vi "Set.vi"(10 "Time Stamp":timestamp, 11 "DateTime in":refnum<class "Timestamp.lvclass">) -> (3 "DateTime out":refnum<class "Timestamp.lvclass">)   [LabVIEW 2022 SP3, in "Conditum.lvlib" / "Columns.lvlib" / "Timestamp.lvclass"]
uses:
  Timestamp.lvclass
  C:/dev/lv/illuminated-g/lv-conditum/Conditum/Columns/Type/Type.lvclass
  Type/Type.lvclass/Type.ctl
  Timestamp.lvclass/Timestamp.ctl
  Type/Type.lvclass
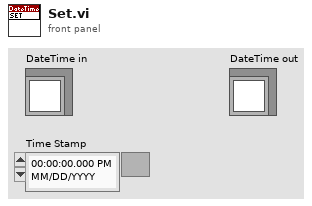
[diagram p1: front panel]
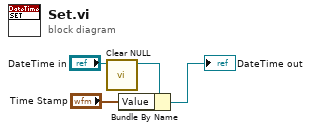
[diagram p0: block diagram]
diagram:
  n1 = call "Clear NULL.vi"("Type in"="DateTime in") -> ("Type out"=w1:refnum<class "Timestamp.lvclass">)  [unwired: 10 in]
  n2 = Bundle By Name(cluster=w1, "Value"="Time Stamp") -> (→"DateTime out":refnum<class "Timestamp.lvclass">)
